vi "Add Depth.vi"(8 "error in (no error)":errorcluster, 10 "Delta Depth":i32, 11 "SnailNum in":refnum<class "SnailNum.lvclass">) -> (0 "error out":errorcluster, 3 "SnailNum out":refnum<class "SnailNum.lvclass">)   [LabVIEW 2020, in "SnailNum.lvclass"]
uses:
  SnailNum.lvclass
  SnailNum.lvclass/SnailNum.ctl
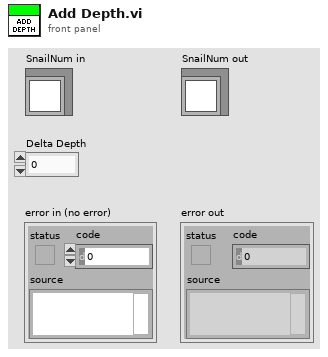
[diagram p1: front panel]
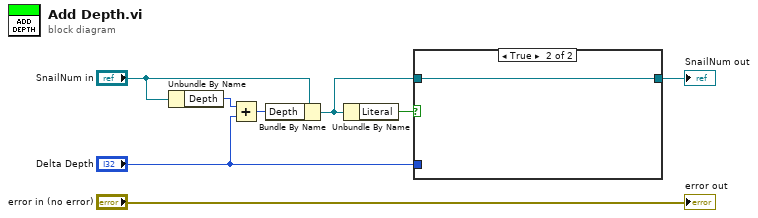
[diagram p0: block diagram]
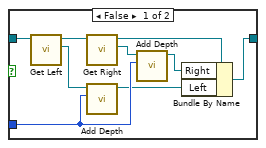
[diagram p2: hidden frame]
diagram:
  n1 = Unbundle By Name("SnailNum in") -> ("Depth"=w7:i32)
  n2 = Add(x=w7, y="Delta Depth") -> (x+y=w5:i32)
  n3 = Bundle By Name(cluster="SnailNum in", "Depth"=w5) -> (w3:refnum<class "SnailNum.lvclass">)
  n4 = Unbundle By Name(w3) -> ("Literal"=w4:bool)
  n5 = case shown="True" w4 {
    tunnel: w3 -> [w17 w18]
    tunnel: [w9 w18] -> w2
    tunnel: "Delta Depth" -> [w13 _]
    frame False {
      n6 = call "Get Left.vi"("SnailNum in"=w17) -> ("Left"=w15:refnum<class "SnailNum.lvclass">, "SnailNum out"=w16:refnum<class "SnailNum.lvclass">)  [unwired: 8 in, 1 out]
      n7 = call "Get Right.vi"("SnailNum in"=w16) -> ("Right"=w14:refnum<class "SnailNum.lvclass">, "SnailNum out"=w12:refnum<class "SnailNum.lvclass">)  [unwired: 8 in, 1 out]
      n8 = call "Add Depth.vi"("Delta Depth"=w13, "SnailNum in"=w15) -> ("SnailNum out"=w11:refnum<class "SnailNum.lvclass">)  [unwired: 8 in, 1 out]
      n9 = call "Add Depth.vi"("Delta Depth"=w13, "SnailNum in"=w14) -> ("SnailNum out"=w10:refnum<class "SnailNum.lvclass">)  [unwired: 8 in, 1 out]
      n10 = Bundle By Name(cluster=w12, "Right"=w10, "Left"=w11) -> (w9:refnum<class "SnailNum.lvclass">)
    }
    frame True {
    }
  }
  "SnailNum out" <- w2
  "error out" <- "error in (no error)"
